vi "Config Type Def to Generic Type Defs.vi"(8 "error in (no error)":errorcluster, 11 "measurement configuration":T12={"digital serial cfg file"="", "digital channel list"="7821\\PCMo 8", "master clock channel list"="7821\\PCMo 0", "output level start"=-1.0, "output level stop"=20.0, "output sweep number of steps"=20000, "output level units"=enum."dBFS", "output range (pk-pk)"=15.0, "load impedance"=4.0, "signal phase"=0.0, "acq sampling rate"=51200.0, "min measurement cycles"=20, "min measurement time (s)"=0.1, "min settling cycles"=0, "min settling time (s)"=0.0, "acq channel"="", "band start"=20.0, "band stop"=20000.0, "weighting filter"=enum."A-weighting", "highpass filter"=enum."DC", "lowpass filter"=enum."No filter", "SNR units"=enum."dB", "THD+N units"=enum."dB", "THD units"=enum."dB", "gain units"=enum."dB", "power measurement method"=enum."DMM", "power measurement resource"="", "power supply voltage"=1.0, "power supply current limit"=0.0, "sense resistor (Ohms)"=0.05} {"min measurement cycles" format="%#_6pHz"; "acq sampling rate" format="%0.2f"}) -> (0 "error out":errorcluster, 3 "single tone settings":T1={"digital channel list"="7821\\PCMo 8", "frame clock rate"=48000.0, "number of channels"=2, "channel length"=32, "bit depth"=24, "data justification"=enum."Left Justified", "endianness"=enum."MSB First", "bit clock edge sync"=enum."Falling", "frame sync edge for channel 0"=enum."Falling", "channel 0 offset"=1, "master clock channel list"="7821\\PCMo 0", "master clock rate"=12288000.0, "enable dither"=TRUE, "logic level"=enum."3.3 V", "signal frequency"=1000.0, "output level"=-1.0, "output level units"=enum."dBFS", "output range (pk-pk)"=15.0, "load impedance"=4.0, "signal phase"=0.0, "acq sampling rate"=51200.0, "min measurement cycles"=20, "min measurement time (s)"=0.1, "min settling cycles"=0, "min settling time (s)"=0.0, "acq channel"="", "band start"=20.0, "band stop"=20000.0, "weighting filter"=enum."A-weighting", "highpass filter"=enum."DC", "lowpass filter"=enum."No filter", "SNR units"=enum."dB", "THD+N units"=enum."dB", "THD units"=enum."dB", "gain units"=enum."dB"} {"signal phase" format="%0.2f"; "master clock rate" format="%#_6pHz"; "frame clock rate" format="%#_6pHz"})   [LabVIEW 2021, in "Noise Sweep_Class D Amplifier.lvlib"]
uses:
  Noise Sweep_Class D Amplifier.lvlib
  Measurement Configuration.ctl
  shared/controls/digital output level units.ctl
  shared/controls/weighting filter.ctl
  shared/controls/highpass filter.ctl
  shared/controls/lowpass filter.ctl
  shared/controls/units - snr.ctl
  shared/controls/units - ratio.ctl
  shared/controls/power measurement method.ctl
  shared/controls/single tone measurement settings (HW).ctl
  shared/controls/digital audio protocol/data justification.ctl
  shared/controls/digital audio protocol/endianness.ctl
  shared/controls/digital audio protocol/digital edge.ctl
  shared/controls/digital audio protocol/logic level.ctl
  shared/controls/audio controls.lvlib
  shared/controls/digital audio protocol/digital audio protocol controls.lvlib
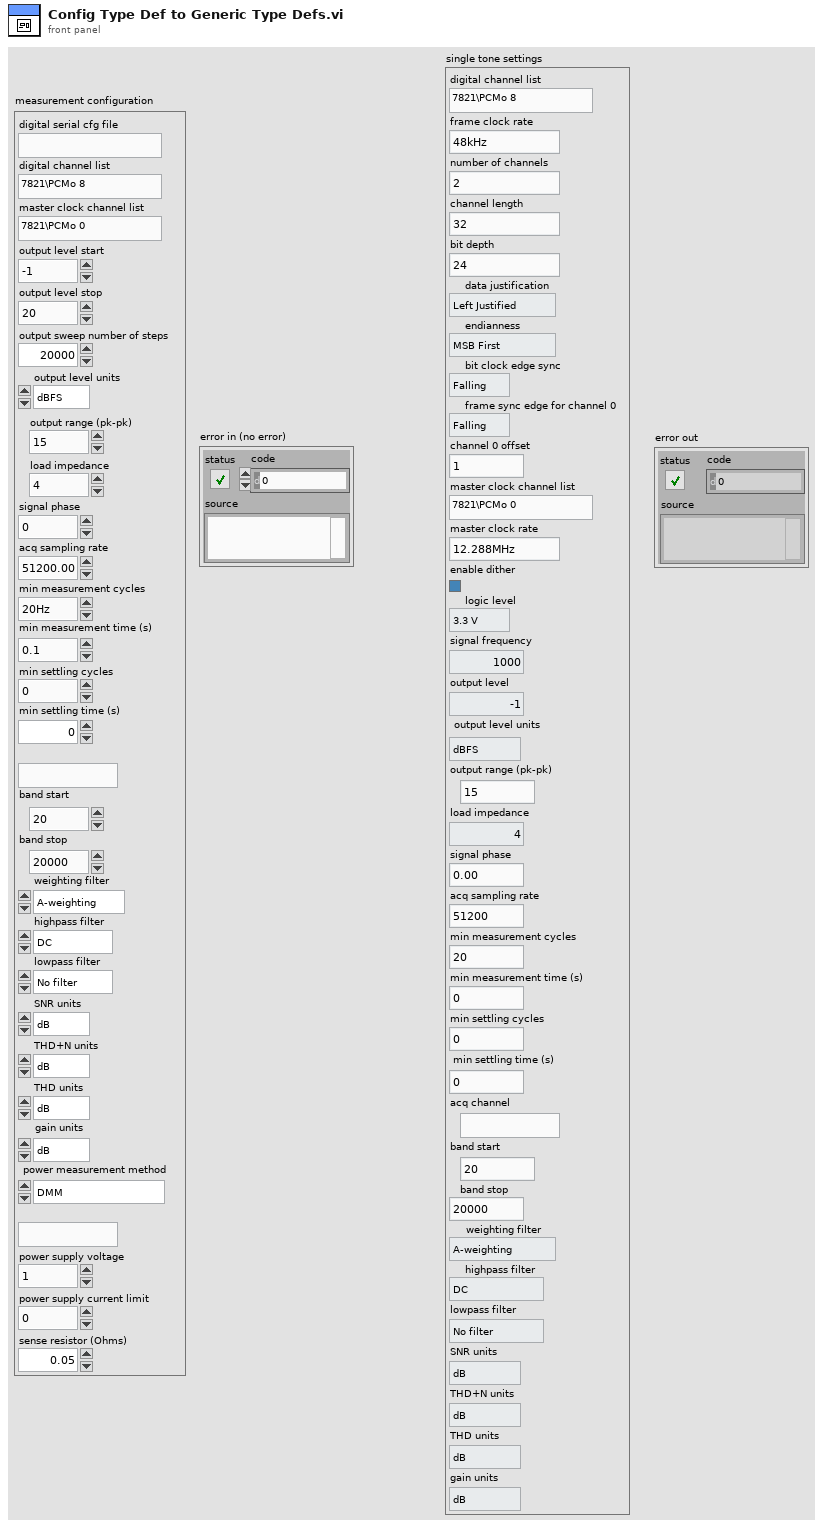
[diagram p1: front panel]
types:
  T1 = typedef "single tone measurement settings (HW).ctl" = cluster{"digital channel list":string, "frame clock rate":dbl, "number of channels":u32, "channel length":u32, "bit depth":u32, "data justification":T2, "endianness":T3, "bit clock edge sync":T4, "frame sync edge for channel 0":T4, "channel 0 offset":u32, "master clock channel list":string, "master clock rate":dbl, "enable dither":bool, "logic level":T5, "signal frequency":dbl, "output level":dbl, "output level units":T6, "output range (pk-pk)":dbl, "load impedance":dbl, "signal phase":dbl, "acq sampling rate":dbl, "min measurement cycles":u32, "min measurement time (s)":dbl, "min settling cycles":u32, "min settling time (s)":dbl, "acq channel":string, "band start":dbl, "band stop":dbl, "weighting filter":T7, "highpass filter":T8, "lowpass filter":T9, "SNR units":T10, "THD+N units":T11, "THD units":T11, "gain units":T11}
  T2 = typedef "data justification.ctl" = enum32{"Left Justified", "Right Justified"}
  T3 = typedef "endianness.ctl" = enum32{"MSB First", "LSB First"}
  T4 = typedef "digital edge.ctl" = enum32{"Rising", "Falling"}
  T5 = typedef "logic level.ctl" = enum32{"3.3 V", "1.8 V", "1.2 V"}
  T6 = typedef "audio controls.lvlib/digital output level units.ctl" = enum32{"% FS", "dBFS", "V"}
  T7 = typedef "weighting filter.ctl" = enum32{"Linear", "A-weighting", "B-weighting", "C-weighting"}
  T8 = typedef "highpass filter.ctl" = enum32{"DC", "AC"}
  T9 = typedef "lowpass filter.ctl" = enum32{"No filter", "AES17 20kHz", "AES17 40kHz"}
  T10 = typedef "audio controls.lvlib/units - snr.ctl" = enum32{"dB", "x/y"}
  T11 = typedef "audio controls.lvlib/units - ratio.ctl" = enum32{"dB", "%", "x/y"}
  T12 = typedef "Noise Sweep_Class D Amplifier.lvlib/Measurement Configuration.ctl" = cluster{"digital serial cfg file":string, "digital channel list":string, "master clock channel list":string, "output level start":dbl, "output level stop":dbl, "output sweep number of steps":u32, "output level units":T6, "output range (pk-pk)":dbl, "load impedance":dbl, "signal phase":dbl, "acq sampling rate":dbl, "min measurement cycles":u32, "min measurement time (s)":dbl, "min settling cycles":u32, "min settling time (s)":dbl, "acq channel":string, "band start":dbl, "band stop":dbl, "weighting filter":T7, "highpass filter":T8, "lowpass filter":T9, "SNR units":T10, "THD+N units":T11, "THD units":T11, "gain units":T11, "power measurement method":T13, "power measurement resource":string, "power supply voltage":dbl, "power supply current limit":dbl, "sense resistor (Ohms)":dbl}
  T13 = typedef "power measurement method.ctl" = enum32{"SMU", "DMM"}
  T14 = typedef "digital audio protocol controls.lvlib/digital audio protocol settings.ctl" = cluster{"number of channels":u32, "data justification":T15, "endianness":T16, "channel length":u32, "bit depth":u32, "frame clock rate":dbl, "bit clock edge sync":T17, "master clock rate":dbl, "Logic Level":T18, "frame sync edge for channel 0":T17, "Channel 0 Offset":u32}
  T15 = typedef "PDM Shared.lvlib/PCM Data Justification.ctl" = enum16{"Left Justified", "Right Justified"}
  T16 = typedef "PDM Shared.lvlib/PCM Bit Endianness.ctl" = enum16{"MSB First", "LSB First"}
  T17 = typedef "PDM Shared.lvlib/Digital Edge.ctl" = enum8{"Rising", "Falling"}
  T18 = typedef "PDM Acquisition Class Library.lvlib/DecoderSession.lvclass/Logic Levels.ctl" = enum16{"3.3 V", "1.8 V", "1.2 V"}
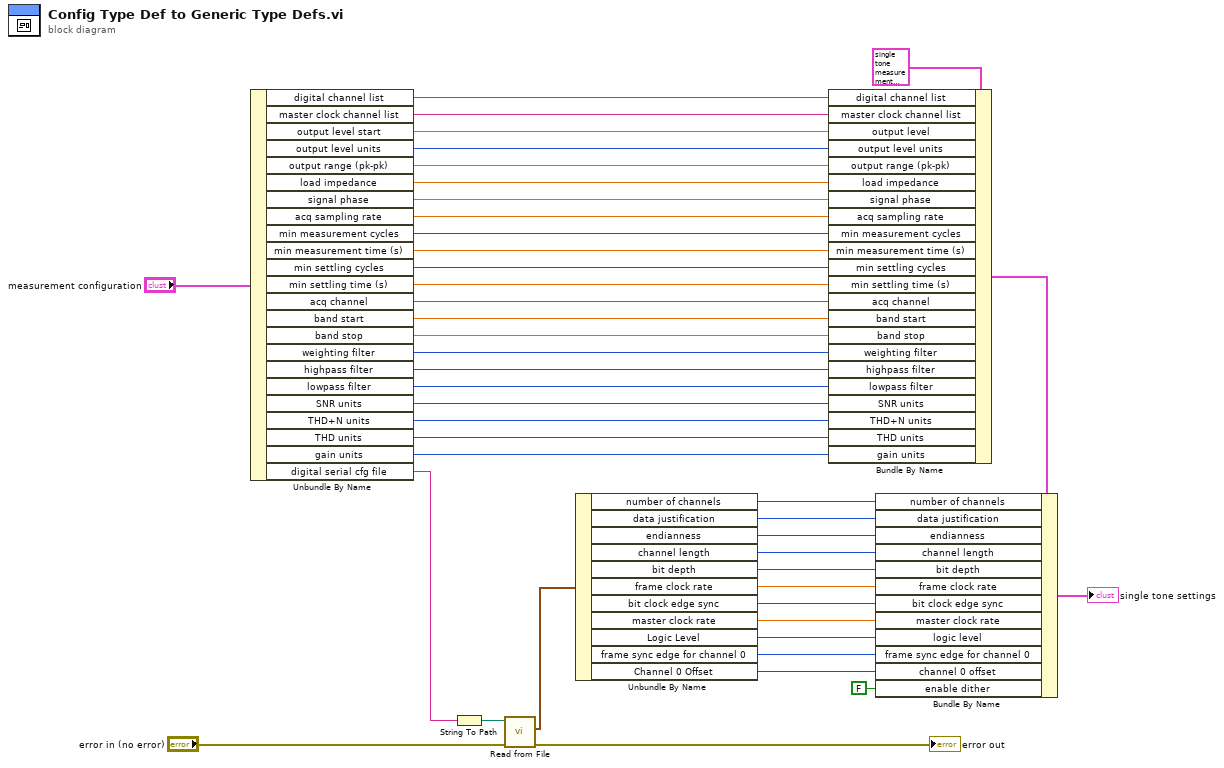
[diagram p0: block diagram]
diagram:
  n1 = Unbundle By Name("measurement configuration") -> ("digital channel list"=w41:string, "master clock channel list"=w40:string, "output level start"=w20:dbl, "output level units"=w39:T6, "output range (pk-pk)"=w38:dbl, "load impedance"=w37:dbl, "signal phase"=w36:dbl, "acq sampling rate"=w35:dbl, "min measurement cycles"=w34:u32, "min measurement time (s)"=w33:dbl, "min settling cycles"=w32:u32, "min settling time (s)"=w31:dbl, "acq channel"=w30:string, "band start"=w29:dbl, "band stop"=w28:dbl, "weighting filter"=w27:T7, "highpass filter"=w26:T8, "lowpass filter"=w25:T9, "SNR units"=w24:T10, "THD+N units"=w23:T11, "THD units"=w22:T11, "gain units"=w21:T11, "digital serial cfg file"=w17:string)
  n2 = String To Path(string=w17) -> (path=w19:path)
  n3 = call "Read from File.vi"("error in (no error)"="error in (no error)", "file path"=w19) -> ("error out"=→"error out":errorcluster, "digital audio protocol settings"=w15:T14)  [unwired: 7 in, 1 out]
  n4 = Unbundle By Name(w15) -> ("number of channels"=w13:u32, "data justification"=w10:T15, "endianness"=w9:T16, "channel length"=w8:u32, "bit depth"=w7:u32, "frame clock rate"=w6:dbl, "bit clock edge sync"=w5:T17, "master clock rate"=w4:dbl, "Logic Level"=w3:T18, "frame sync edge for channel 0"=w2:T17, "Channel 0 Offset"=w1:u32)
  n5 = Bundle By Name(cluster=T1 {"digital channel list"="7821\\PCMo 8", "frame clock rate"=48000.0, "number of channels"=2, "channel length"=32, "bit depth"=24, "data justification"=enum."Left Justified", "endianness"=enum."MSB First", "bit clock edge sync"=enum."Falling", "frame sync edge for channel 0"=enum."Falling", "channel 0 offset"=1, "master clock channel list"="7821\\PCMo 0", "master clock rate"=12288000.0, "enable dither"=TRUE, "logic level"=enum."3.3 V", "signal frequency"=1000.0, "output level"=-1.0, "output level units"=enum."dBFS", "output range (pk-pk)"=15.0, "load impedance"=4.0, "signal phase"=0.0, "acq sampling rate"=51200.0, "min measurement cycles"=20, "min measurement time (s)"=0.1, "min settling cycles"=0, "min settling time (s)"=0.0, "acq channel"="", "band start"=20.0, "band stop"=20000.0, "weighting filter"=enum."A-weighting", "highpass filter"=enum."DC", "lowpass filter"=enum."No filter", "SNR units"=enum."dB", "THD+N units"=enum."dB", "THD units"=enum."dB", "gain units"=enum."dB"} ("measurement configuration"), "digital channel list"=w41, "master clock channel list"=w40, "output level"=w20, "output level units"=w39, "output range (pk-pk)"=w38, "load impedance"=w37, "signal phase"=w36, "acq sampling rate"=w35, "min measurement cycles"=w34, "min measurement time (s)"=w33, "min settling cycles"=w32, "min settling time (s)"=w31, "acq channel"=w30, "band start"=w29, "band stop"=w28, "weighting filter"=w27, "highpass filter"=w26, "lowpass filter"=w25, "SNR units"=w24, "THD+N units"=w23, "THD units"=w22, "gain units"=w21) -> (w14:T1)
  n6 = Bundle By Name(cluster=w14, "number of channels"=w13, "data justification"=w10, "endianness"=w9, "channel length"=w8, "bit depth"=w7, "frame clock rate"=w6, "bit clock edge sync"=w5, "master clock rate"=w4, "logic level"=w3, "frame sync edge for channel 0"=w2, "channel 0 offset"=w1, "enable dither"=FALSE) -> (→"single tone settings":T1)
